vi "GetAllPosts.vi"(8 "error in (no error)":errorcluster, 11 "ErrorManager in":refnum<class "ErrorManager.lvclass">) -> (0 "error out":errorcluster, 1 "Errors":T1[](array[typedef]), 3 "ErrorManager out":refnum<class "ErrorManager.lvclass">)   [LabVIEW 2020, in "ErrorManager.lvlib" / "ErrorManager.lvclass"]
uses:
  ErrorManager.lvclass
  ErrorInfo.ctl
  ErrorType.ctl
  ErrorManager.lvclass/ErrorManager.ctl
  LabVIEWObjectInterfaces/IErrorManager/IErrorManager.lvclass
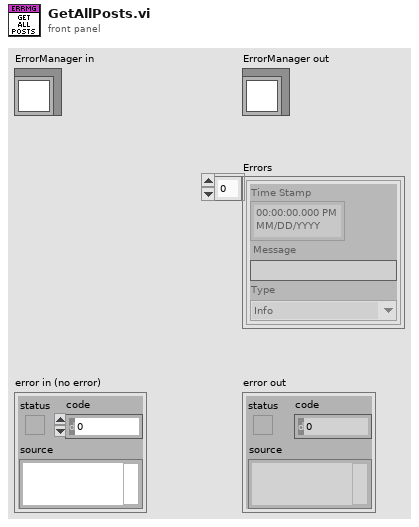
[diagram p1: front panel]
types:
  T1 = typedef "ErrorManager.lvlib/ErrorManager.lvclass/ErrorInfo.ctl" = cluster{"Time Stamp":timestamp, "Message":string, "Type":T2}
  T2 = typedef "LabVIEWObjectInterfaces.lvlib/IErrorManager.lvclass/ErrorType.ctl" = enum16{"Info", "Warning", "Error"}
  T3 = typedef "ErrorManager.lvlib/ErrorManager.lvclass/ErrorInfoArrayRef.ctl" = refnum<data-value>
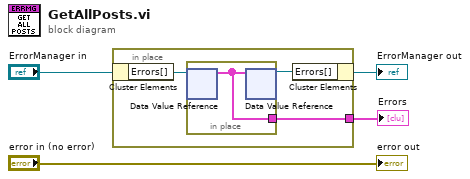
[diagram p0: block diagram]
diagram:
  n1 = in-place {
    in-place-border: [w5] -> w1
    n2 = in-place-cluster #1("ErrorManager in") -> ("Errors[]"=w7:T3)
    n3 = in-place {
      in-place-border: [w8] -> w5
      n4 = in-place-dvr #2(w7) -> (w8:T1[])  [unwired: 1 out]
      n5 = in-place-dvr #2(w8) -> (w6:T3)  [unwired: 1 out]
    }
    n6 = in-place-cluster #1("Errors[]"=w6) -> (→"ErrorManager out":refnum<class "ErrorManager.lvclass">)
  }
  "Errors" <- w1
  "error out" <- "error in (no error)"
